vi "Disabled.vi"(7 "Robot Mode":T2, 10 "Match Info":T1={"Autonomous Elapsed Seconds"=0.0, "TeleOp Elapsed Seconds"=0.0, "Disabled Elapsed Seconds"=0.0, "Visited Autonomous"=FALSE, "Visited TeleOp"=FALSE, "Visited Disabled"=FALSE, "Autonomous Settings"={"Autonomous Style"=enum."Independent", "VI Refnum"=refnum}}, 11 "Call Context":T3) -> ()   [LabVIEW 2011]
doc: "This VI is called each time a disabled packet is received from the DS. It is often used to prepare for the next robot mode, to calibrate sensors, etc."
uses:
  <vilib>/Rock Robotics/WPI/DriverStation/WPI_DriverStationDerivedRobotMode.ctl
  <vilib>/Rock Robotics/WPI/DriverStation/WPI_DriverStationRobotMode.ctl
  <vilib>/Rock Robotics/WPI/DriverStation/WPI_DriverStationMatch Info.ctl
  Robot Global Data.vi
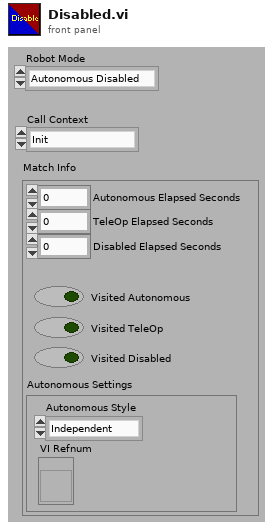
[diagram p1: front panel]
types:
  T1 = typedef "WPI_DriverStationMatch Info.ctl" = cluster{"Autonomous Elapsed Seconds":dbl, "TeleOp Elapsed Seconds":dbl, "Disabled Elapsed Seconds":dbl, "Visited Autonomous":bool, "Visited TeleOp":bool, "Visited Disabled":bool, "Autonomous Settings":cluster{"Autonomous Style":enum16{"Iterative", "Independent"}, "VI Refnum":refnum<vi>}}
  T2 = typedef "WPI_DriverStationRobotMode.ctl" = enum16{"Autonomous Disabled", "Autonomous Enabled", "Teleop Disabled", "Teleop Enabled", "Timeout", "Finish"}
  T3 = typedef "WPI_DriverStationDerivedRobotMode.ctl" = enum16{"Init", "Execute", "Stop"}
  T4 = typedef "WPI_JoystickDevRef.ctl" = cluster{"Device":T5}
  T5 = typedef "WPI_JoystickDeviceEnum.ctl" = enum16{"USB 1", "USB 2", "USB 3", "USB 4", "Kinect 1", "Kinect 2"}
  T6 = typedef "WPI_JoystickButtonState.ctl" = cluster{"Button 1":bool, "Button 2":bool, "Button 3":bool, "Button 4":bool, "Button 5":bool, "Button 6":bool, "Button 7":bool, "Button 8":bool, "Button 9":bool, "Button 10":bool, "Button 11":bool, "Button 12":bool}
  T7 = typedef "WPI_MotorControlDeviceRef.ctl" = cluster{"DeviceStatus":errorcluster, "Type":enum16{"PWM", "CAN"}, "PWM":cluster{"Digital Module":T8, "PWM Channel":T9, "DeadBand":T10}, "CAN":cluster{"Device Number":u8, "Control Mode":T11, "Semaphore":T12, "Max Vout":dbl}, "Invert":bool, "TransformRef":T13, "InvTransformRef":T13}
  T8 = typedef "FPGA_TypedefDigitalModule.ctl" = enum16{"Digital Module 1", "Digital Module 2"}
  T9 = typedef "FPGA_DIOPWMChannel.ctl" = enum8{"PWM 1", "PWM 2", "PWM 3", "PWM 4", "PWM 5", "PWM 6", "PWM 7", "PWM 8", "PWM 9", "PWM 10", "Invalid"}
  T10 = typedef "WPI_PWMDeadband.ctl" = cluster{"Name":string, "maxPositivePwm":i32, "minPositivePwm":i32, "centerPwm":i32, "maxNegativePwm":i32, "minNegativePwm":i32, "angularRange":u16}
  T11 = typedef "WPI_CANJaguar_ControlMode.ctl" = enum8{"Percent VBus", "Current", "Speed", "Position", "Voltage"}
  T12 = typedef "Semaphore RefNum" = refnum<k1>
  T13 = typedef "WPI_PWMTransform_ConPane.ctl" = refnum<vi>
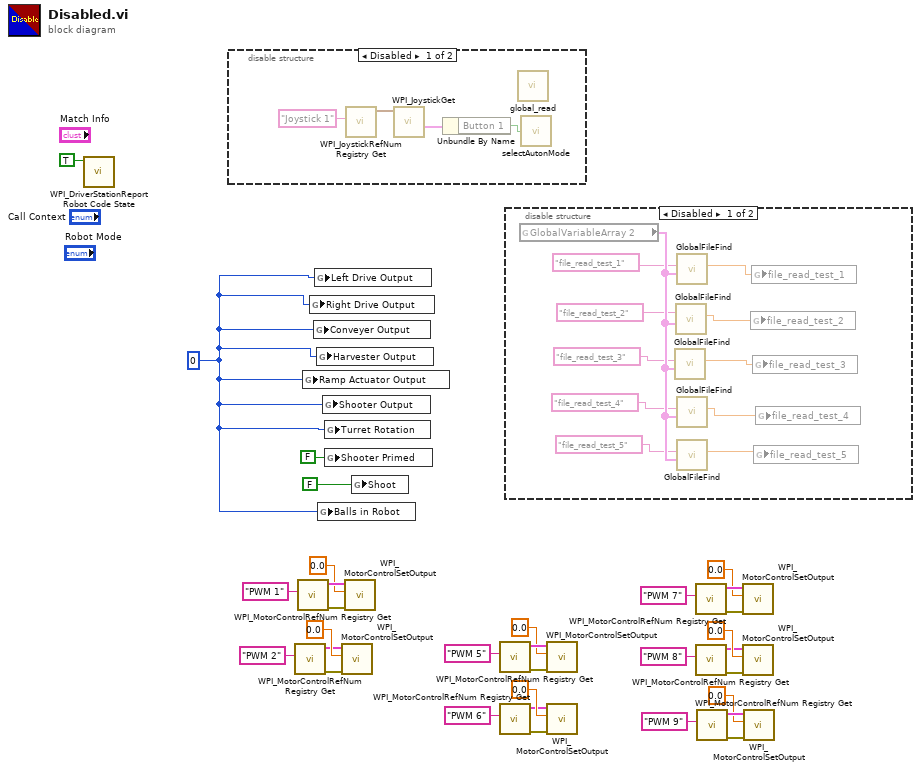
[diagram p0: block diagram]
diagram:
  w1 = 0
  n1 = call <vilib>:"WPI_DriverStationReport Robot Code State.vi"("Disabled"=TRUE ("Autonomous")) -> ()  [unwired: 10 in, 1 out]
  n2 = disable-structure shown="Disabled" {
    frame Disabled {
      n3 = call <vilib>:"WPI_JoystickRefNum Registry Get.vi"("refnum name"="Joystick 1") -> ("JoystickDevRef"=w35:T4)  [unwired: 9 in, 1 out]
      n4 = call <vilib>:"WPI_JoystickGet.vi"("JoystickDevRef"=w35) -> ("Buttons"=w34:T6)  [unwired: 4 in, 2 out]
      n5 = Unbundle By Name(w34) -> ("Button 1"=w33:bool)
      n6 = call "global_read.vi"() -> ()  [unwired: 12 in]
      n7 = call "selectAutonMode.vi"("Joystick"=w33) -> ()  [unwired: 1 in]
    }
    frame Enabled {
    }
  }
  n8 = call <vilib>:"WPI_MotorControlRefNum Registry Get.vi"("refnum name"="PWM 2") -> ("error out"=w25:errorcluster, "MotorControlDevRef"=w24:T7)  [unwired: 9 in]
  n9 = call <vilib>:"WPI_MotorControlRefNum Registry Get.vi"("refnum name"="PWM 1") -> ("error out"=w30:errorcluster, "MotorControlDevRef"=w31:T7)  [unwired: 9 in]
  n10 = global write "Robot Global Data.vi" "Ramp Actuator Output"(w1) -> ()
  n11 = global write "Robot Global Data.vi" "Right Drive Output"(w1) -> ()
  n12 = global write "Robot Global Data.vi" "Conveyer Output"(w1) -> ()
  n13 = global write "Robot Global Data.vi" "Left Drive Output"(w1) -> ()
  n14 = global write "Robot Global Data.vi" "Harvester Output"(w1) -> ()
  n15 = global write "Robot Global Data.vi" "Balls in Robot"(w1) -> ()
  n16 = global write "Robot Global Data.vi" "Shooter Output"(w1) -> ()
  n17 = global write "Robot Global Data.vi" "Turret Rotation"(w1) -> ()
  n18 = global write "Robot Global Data.vi" "Shooter Primed"(FALSE ("Shooter Primed")) -> ()
  n19 = call <vilib>:"WPI_MotorControlSetOutput.vi"("error in (no error)"=w25, "Output"=0.0, "MotorControlDevRef"=w24) -> ()  [unwired: 7 in, 2 out]
  n20 = call <vilib>:"WPI_MotorControlSetOutput.vi"("error in (no error)"=w30, "Output"=0.0, "MotorControlDevRef"=w31) -> ()  [unwired: 7 in, 2 out]
  n21 = global write "Robot Global Data.vi" "Shoot"(FALSE ("Shooter Primed")) -> ()
  n22 = call <vilib>:"WPI_MotorControlRefNum Registry Get.vi"("refnum name"="PWM 5") -> ("error out"=w22:errorcluster, "MotorControlDevRef"=w23:T7)  [unwired: 9 in]
  n23 = call <vilib>:"WPI_MotorControlRefNum Registry Get.vi"("refnum name"="PWM 6") -> ("error out"=w17:errorcluster, "MotorControlDevRef"=w16:T7)  [unwired: 9 in]
  n24 = disable-structure shown="Disabled" {
    frame Disabled {
      n25 = global read "Robot Global Data.vi" "GlobalVariableArray 2"() -> (w47:cluster{"name":string, "va;":dbl}[])
      n26 = call "GlobalFileFind.vi"("GlobalVariableArray 2"=w47, "VariableNameLookup"="file_read_test_3") -> ("VariableValueOut"=w38:dbl)  [unwired: 9 in]
      n27 = call "GlobalFileFind.vi"("GlobalVariableArray 2"=w47, "VariableNameLookup"="file_read_test_2") -> ("VariableValueOut"=w37:dbl)  [unwired: 9 in]
      n28 = call "GlobalFileFind.vi"("GlobalVariableArray 2"=w47, "VariableNameLookup"="file_read_test_1") -> ("VariableValueOut"=w41:dbl)  [unwired: 9 in]
      n29 = call "GlobalFileFind.vi"("GlobalVariableArray 2"=w47, "VariableNameLookup"="file_read_test_4") -> ("VariableValueOut"=w39:dbl)  [unwired: 9 in]
      n30 = call "GlobalFileFind.vi"("GlobalVariableArray 2"=w47, "VariableNameLookup"="file_read_test_5") -> ("VariableValueOut"=w40:dbl)  [unwired: 9 in]
      n31 = global write "Robot Global Data.vi" "file_read_test_2"(w37) -> ()
      n32 = global write "Robot Global Data.vi" "file_read_test_1"(w41) -> ()
      n33 = global write "Robot Global Data.vi" "file_read_test_3"(w38) -> ()
      n34 = global write "Robot Global Data.vi" "file_read_test_5"(w40) -> ()
      n35 = global write "Robot Global Data.vi" "file_read_test_4"(w39) -> ()
    }
    frame Enabled {
    }
  }
  n36 = call <vilib>:"WPI_MotorControlSetOutput.vi"("error in (no error)"=w22, "Output"=0.0, "MotorControlDevRef"=w23) -> ()  [unwired: 7 in, 2 out]
  n37 = call <vilib>:"WPI_MotorControlSetOutput.vi"("error in (no error)"=w17, "Output"=0.0, "MotorControlDevRef"=w16) -> ()  [unwired: 7 in, 2 out]
  n38 = call <vilib>:"WPI_MotorControlRefNum Registry Get.vi"("refnum name"="PWM 7") -> ("error out"=w14:errorcluster, "MotorControlDevRef"=w15:T7)  [unwired: 9 in]
  n39 = call <vilib>:"WPI_MotorControlRefNum Registry Get.vi"("refnum name"="PWM 8") -> ("error out"=w9:errorcluster, "MotorControlDevRef"=w8:T7)  [unwired: 9 in]
  n40 = call <vilib>:"WPI_MotorControlRefNum Registry Get.vi"("refnum name"="PWM 9") -> ("error out"=w6:errorcluster, "MotorControlDevRef"=w7:T7)  [unwired: 9 in]
  n41 = call <vilib>:"WPI_MotorControlSetOutput.vi"("error in (no error)"=w14, "Output"=0.0, "MotorControlDevRef"=w15) -> ()  [unwired: 7 in, 2 out]
  n42 = call <vilib>:"WPI_MotorControlSetOutput.vi"("error in (no error)"=w9, "Output"=0.0, "MotorControlDevRef"=w8) -> ()  [unwired: 7 in, 2 out]
  n43 = call <vilib>:"WPI_MotorControlSetOutput.vi"("error in (no error)"=w6, "Output"=0.0, "MotorControlDevRef"=w7) -> ()  [unwired: 7 in, 2 out]
